vi "Paint_Center_of_Particle-8.vi"(0 "[IN] Initialized Image":T4, 1 "[IN] AVI Refnum":T3, 3 "[IN] Image Type":T2 items=["Grayscale (U8)", "Grayscale (I16)", "Grayscale (SGL)", "Complex (CSG)", "RGB (U32)", "HSL (U32)", "RGB (U64)", "Grayscale (U16)"], 5 "[IN] Frame Number":u32, 9 "[IN] Array of X,Y":dbl[](array[numeric]), 11 "error IN":errorcluster, 12 "[IN] Image Filtering Settings":T1, 13 "Keep Nega-\ntive Values?":bool) -> (4 "[OUT] Image Dst":T4, 15 "error OUT":errorcluster)   [LabVIEW 2017]
doc: "SubVI make a picture of all localized particles in a frame\nCrosses - centers of particles"
uses:
  <vilib>/vision/Image Controls.llb/IMAQ Image.ctl
  <vilib>/vision/Avi.llb/IMAQ AVI2 Refnum.ctl
  <vilib>/vision/NI_Vision_Development_Module.lvlib
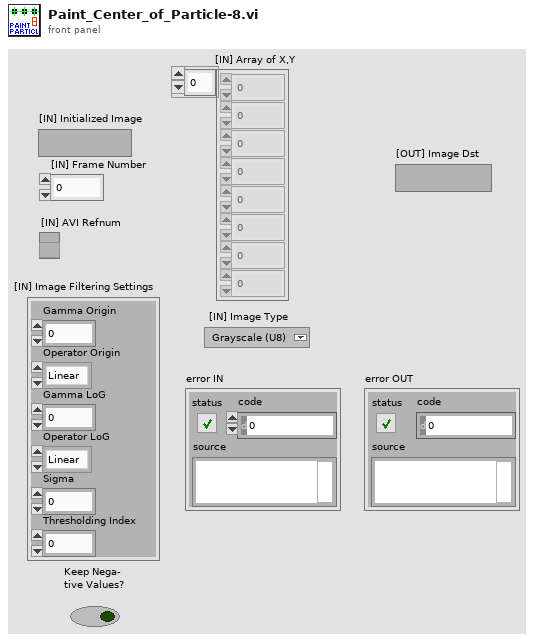
[diagram p1: front panel]
types:
  T1 = cluster{"Gamma Origin":sgl, "Operator Origin":enum32{"Linear", "Log", "Exp", "Square", "Square root", "Power X", "Power 1/X"}, "Gamma LoG":sgl, "Operator LoG":enum32{"Linear", "Log", "Exp", "Square", "Square root", "Power X", "Power 1/X"}, "Sigma":dbl, "Thresholding Index":i8}
  T2 = typedef "Image Type" = u32
  T3 = typedef "IMAQ AVI2 Refnum.ctl" = refnum<k20>
  T4 = typedef "IMAQ Image.ctl" = refnum<image>
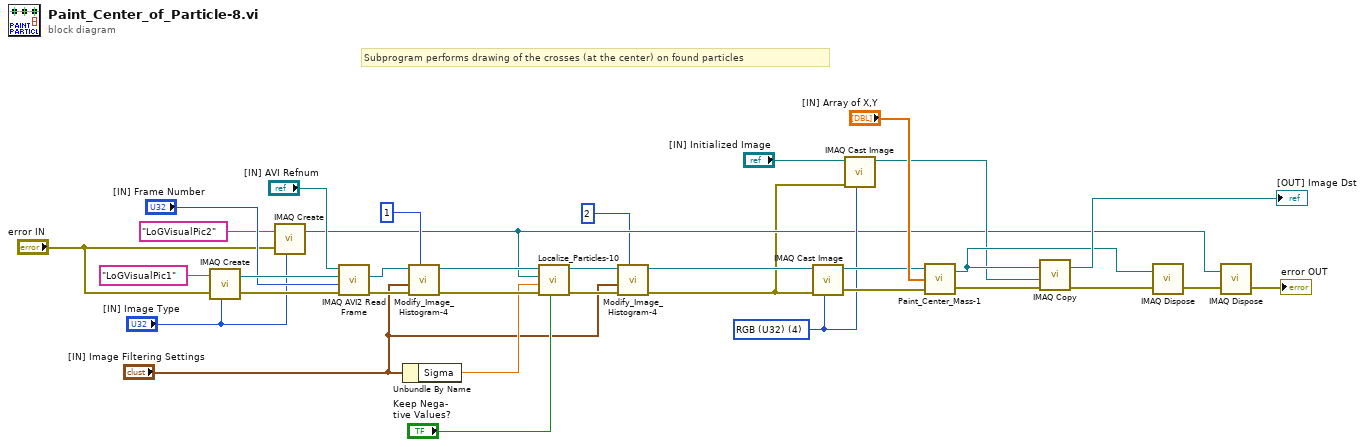
[diagram p0: block diagram]
diagram:
  w19 = T2 4 items=["Grayscale (U8)", "Grayscale (I16)", "Grayscale (SGL)", "Complex (CSG)", "RGB (U32)", "HSL (U32)", "RGB (U64)", "Grayscale (U16)"] ("Image Type")
  # "Subprogram performs drawing of the crosses (at the center) on found particles"
  n1 = call "IMAQ Create"("Image Name"="LoGVisualPic1", "Image Type"="[IN] Image Type", "error in (no error)"="error IN") -> ("New Image"=w32:T4, "error out"=w31:errorcluster)  [unwired: 2 in]
  n2 = call "IMAQ Create"("Image Name"="LoGVisualPic2", "Image Type"="[IN] Image Type", "error in (no error)"="error IN") -> ("New Image"=w9:T4)  [unwired: 2 in, 1 out]
  n3 = call "IMAQ AVI2 Read Frame"("error in (no error)"=w31, "Frame Number"="[IN] Frame Number", "Image"=w32, "AVI Refnum"="[IN] AVI Refnum") -> ("error out"=w12:errorcluster, "Image Out"=w14:T4)  [unwired: 5 in, 1 out]
  n4 = Unbundle By Name("[IN] Image Filtering Settings") -> ("Sigma"=w8:dbl)
  n5 = call "Modify_Image_Histogram-4.vi"("1 - Origin\n2 - LoG"=u8 1 ("1 - Origin\n2 - LoG"), "error IN"=w12, "[IN] Image Filtering Settings"="[IN] Image Filtering Settings", "[IN] LoG Processed Image"=w14) -> ("error OUT"=w10:errorcluster, "[OUT] Histogram Modified Image"=w11:T4)  [unwired: 5 in, 1 out]
  n6 = call "Localize_Particles-10.vi"("Keep Nega-\ntive Values?"="Keep Nega-\ntive Values?", "error IN"=w10, "[IN] Sigma"=w8, "[IN] Destination Image"=w9, "[IN] Frame"=w11) -> ("error OUT"=w5:errorcluster, "[OUT] LoG Processed Image"=w6:T4)  [unwired: 3 in, 1 out]
  n7 = call "Modify_Image_Histogram-4.vi"("1 - Origin\n2 - LoG"=u8 2 ("1 - Origin\n2 - LoG"), "error IN"=w5, "[IN] Image Filtering Settings"="[IN] Image Filtering Settings", "[IN] LoG Processed Image"=w6) -> ("error OUT"=w1:errorcluster, "[OUT] Histogram Modified Image"=w2:T4)  [unwired: 5 in, 1 out]
  n8 = call "IMAQ Cast Image"("Image Type"=w19, "error in (no error)"=w1, "Image Src"=w2) -> ("error out"=w21:errorcluster, "Image Dst Out"=w22:T4)  [unwired: 7 in]
  n9 = call "IMAQ Cast Image"("Image Type"=w19, "error in (no error)"=w1, "Image Src"="[IN] Initialized Image") -> ("Image Dst Out"=w18:T4)  [unwired: 7 in, 1 out]
  n10 = call "Paint_Center_Mass-1.vi"("error IN"=w21, "Array of Points IN"="[IN] Array of X,Y", "Image IN"=w22) -> ("error OUT"=w27:errorcluster, "Image OUT"=w26:T4)
  n11 = call "IMAQ Copy"("error in (no error)"=w27, "Image Dst"=w18, "Image Src"=w26) -> ("error out"=w30:errorcluster, "Image Dst Out"=→"[OUT] Image Dst":T4)  [unwired: 3 in]
  n12 = call "IMAQ Dispose"("Image"=w26, "error in (no error)"=w30) -> ("error out"=w17:errorcluster)  [unwired: 4 in]
  n13 = call "IMAQ Dispose"("Image"=w9, "error in (no error)"=w17) -> ("error out"=→"error OUT":errorcluster)  [unwired: 4 in]
